vi "Manipulate_Theta.vi"(8 "error in (no error)":errorcluster, 11 "Theta in":dbl) -> (0 "error out":errorcluster, 2 "Boolean":bool, 3 "Theta out":dbl)   [LabVIEW 2017]
doc: "Perform manipulations to Theta based on flags. 'Normal Theta' will be true if Theta is decreasing (i.e. direction is towards the destination). 'Swapped Yet' will be true once the 'Normal Theta' flag is flipped to be False."
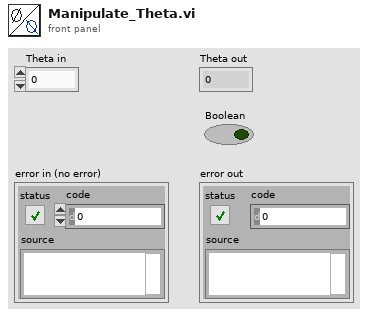
[diagram p1: front panel]
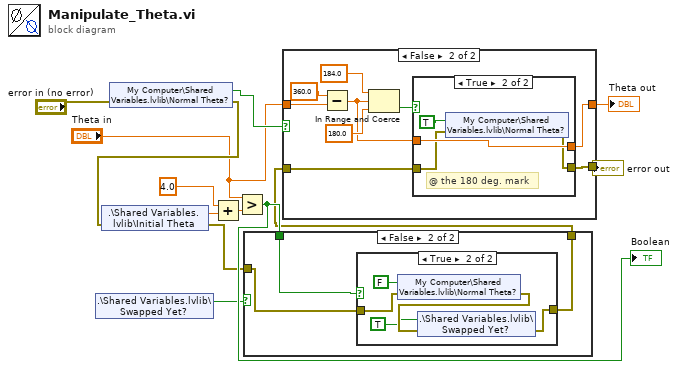
[diagram p0: block diagram]
diagram:
  n1 = shared-variable ".\\Shared Variables.lvlib\\Swapped Yet?"() -> (w9:bool)  [unwired: 1 in, 1 out]
  n2 = shared-variable "My Computer\\Shared Variables.lvlib\\Normal Theta?"(error in="error in (no error)") -> (w7:bool, error out=w6:errorcluster)
  n3 = shared-variable ".\\Shared Variables.lvlib\\Initial Theta"(error in=w6) -> (w12:dbl, error out=w4:errorcluster)
  n4 = Add(x=4.0, y=w12) -> (x+y=w10:dbl)
  n5 = Greater?(x="Theta in", y=w10) -> (0:w13:bool)
  "Boolean" <- w13
  n6 = case shown="False" w9 {
    tunnel: w13 -> [_ w17]
    tunnel: w4 -> [w14 w16]
    tunnel: [w14 w15] -> w8
    frame True {
    }
    frame False {
      n7 = case shown="True" w17 {
        tunnel: w16 -> [w18 w22]
        tunnel: [w18 w20] -> w15
        frame False {
        }
        frame True {
          n8 = shared-variable "My Computer\\Shared Variables.lvlib\\Normal Theta?"(FALSE ("Normal Theta"), error in=w22) -> (error out=w21:errorcluster)
          n9 = shared-variable ".\\Shared Variables.lvlib\\Swapped Yet?"(TRUE ("Swapped Yet?"), error in=w21) -> (error out=w20:errorcluster)
        }
      }
    }
  }
  n10 = case shown="False" w7 {
    tunnel: "Theta in" -> [w25 w34]
    tunnel: [w25 w28] -> w2
    tunnel: w8 -> [w24 w29]
    tunnel: [w24 w27] -> w3
    frame True {
    }
    frame False {
      n11 = Subtract(x=360.0, y=w34) -> (x-y=w30:dbl)
      n12 = In Range and Coerce(upper limit=184.0, x=w30, lower limit=180.0) -> (In Range?=w26:bool)  [unwired: 1 out]
      n13 = case shown="True" w26 {
        tunnel: w30 -> [w36 w40]
        tunnel: [w36 w40] -> w28
        tunnel: w29 -> [w35 w38]
        tunnel: [w35 w37] -> w27
        frame False {
        }
        frame True {
          # "@ the 180 deg. mark"
          n14 = shared-variable "My Computer\\Shared Variables.lvlib\\Normal Theta?"(TRUE ("Normal Theta"), error in=w38) -> (error out=w37:errorcluster)
        }
      }
    }
  }
  "error out" <- w3
  "Theta out" <- w2
